vi "PH_ForceSensor.ProcEvents.vi"(0 "i ref in":refnum<vi>, 5 "error in (no error)":errorcluster) -> (14 "i ref out":refnum<vi>, 19 "error out":errorcluster)   [LabVIEW 2014, in "PH_ForceSensor.lvlib"]
doc: "This method is used to define the events the object will listen to. Add your own events here."
uses:
  PH_ForceSensor.lvlib
  CSCore/BaseProcess/BaseProcess.event definition.ctl
  CSCore/CAEObj/CAEObj.event definition.ctl
  CSCore/BaseProcess/BaseProcess.descriptor string definition.ctl
  PH_Beckhoff_StepMot/PH_Beckhoff_StepMot.Force Sensor Tags.ctl
  PH_Beckhoff_StepMot/PH_Beckhoff_StepMot.Force Sensor Location.ctl
  CSCore/BaseProcess/BaseProcess.lvlib
  CSCore/CAEObj/CAEObj.lvlib
  PH_Common/PH_Common.lvlib
  PH_Beckhoff_StepMot/PH_Beckhoff_StepMot.lvlib
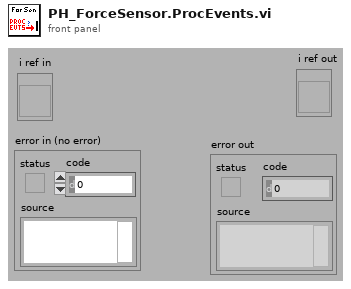
[diagram p1: front panel]
types:
  T1 = typedef "BaseProcess.lvlib/BaseProcess.event definition.ctl" = cluster{"CAEEvtDef":T2, "Data Descriptor":T3}
  T2 = typedef "CAEObj.lvlib/CAEObj.event definition.ctl" = cluster{"URL":string, "enable":bool, "ignoreResID":bool}
  T3 = typedef "BaseProcess.lvlib/BaseProcess.descriptor string definition.ctl" = string
  T4 = typedef "PH_Beckhoff_StepMot.lvlib/PH_Beckhoff_StepMot.Force Sensor Location.ctl" = enum16{"no Info", "MM1"}
  T5 = typedef "PH_Beckhoff_StepMot.lvlib/PH_Beckhoff_StepMot.Force Sensor Tags.ctl" = enum16{"top-front", "top-back", "bottom-front", "bottom-back"}
  T6 = typedef "PH_Common.lvlib/PH_DIM.Event Declarer.ctl" = cluster{"Service Name":string, "Selector":string}
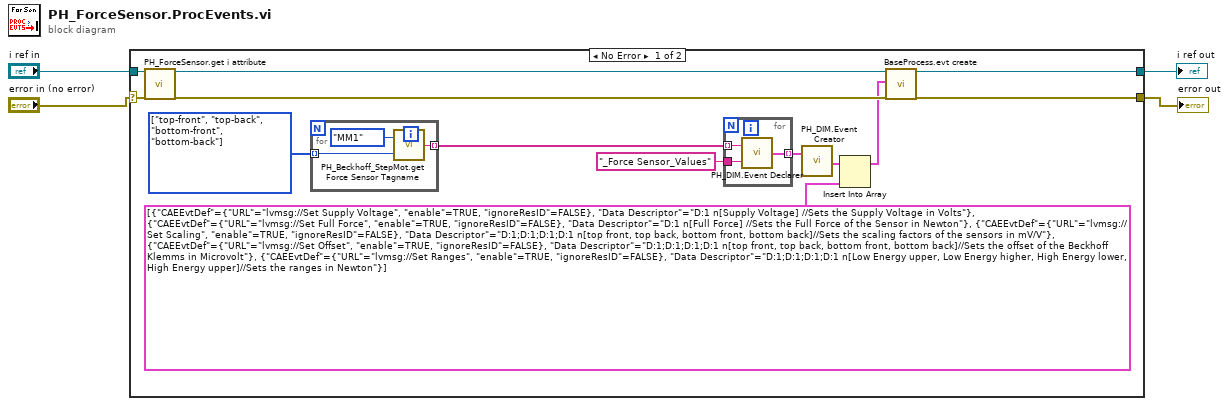
[diagram p0: block diagram]
diagram:
  n1 = case shown="No Error" "error in (no error)" {
    selector: "error in (no error)" -> [w9 w24]
    tunnel: "i ref in" -> [w17 w25]
    tunnel: [w14 w24] -> w3
    tunnel: [w13 w25] -> w2
    frame No Error {
      w7 = T5[] [enum."top-front", enum."top-back", enum."bottom-front", enum."bottom-back"] items=["top-front", "top-back", "bottom-front", "bottom-back"]
      n2 = call "PH_ForceSensor.get i attribute.vi"("i ref in"=w17, "error in (no error)"=w9) -> ("i ref out"=w15:refnum<vi>, "error out"=w16:errorcluster)  [unwired: 15 in, 1 out]
      n3 = for {
        tunnel: w7 -> [w20] mode=indexing
        tunnel: [w18] -> w6 mode=indexing
        n4 = call "PH_Beckhoff_StepMot.get Force Sensor Tagname.vi"("Force Sensor Tag"=w20, "Force Sensor Location"=PH_Beckhoff_StepMot.Force_Sensor_Location."MM1") -> ("Force Sensor Tagname"=w18:string)
      }
      n5 = for {
        tunnel: [w23] -> w12 mode=indexing
        tunnel: "_Force Sensor_Values" -> [w22]
        tunnel: w6 -> [w21] mode=indexing
        n6 = call "PH_DIM.Event Declarer.vi"("Selector"=w22, "Service Name"=w21) -> ("declared DIM Event"=w23:T6)
      }
      n7 = call "PH_DIM.Event Creator.vi"("Trendmessage Services"=w12) -> ("DIM Service Events"=w11:T1[])  [unwired: 18 in]
      n8 = Insert Into Array(array=w11, new element=T1[] [{"CAEEvtDef"={"URL"="lvmsg://Set Supply Voltage", "enable"=TRUE, "ignoreResID"=FALSE}, "Data Descriptor"="D:1 n[Supply Voltage] //Sets the Supply Voltage in Volts"}, {"CAEEvtDef"={"URL"="lvmsg://Set Full Force", "enable"=TRUE, "ignoreResID"=FALSE}, "Data Descriptor"="D:1 n[Full Force] //Sets the Full Force of the Sensor in Newton"}, {"CAEEvtDef"={"URL"="lvmsg://Set Scaling", "enable"=TRUE, "ignoreResID"=FALSE}, "Data Descriptor"="D:1;D:1;D:1;D:1 n[top front, top back, bottom front, bottom back]//Sets the scaling factors of the sensors in mV/V"}, {"CAEEvtDef"={"URL"="lvmsg://Set Offset", "enable"=TRUE, "ignoreResID"=FALSE}, "Data Descriptor"="D:1;D:1;D:1;D:1 n[top front, top back, bottom front, bottom back]//Sets the offset of the Beckhoff Klemms in Microvolt"}, {"CAEEvtDef"={"URL"="lvmsg://Set Ranges", "enable"=TRUE, "ignoreResID"=FALSE}, "Data Descriptor"="D:1;D:1;D:1;D:1 n[Low Energy upper, Low Energy higher, High Energy lower, High Energy upper]//Sets the ranges in Newton"}] ("new events")) -> (w10:T1[])  [unwired: 1 in]
      n9 = call "BaseProcess.evt create.vi"("i ref in"=w15, "newEvents"=w10, "error in (no error)"=w16) -> ("i ref out"=w13:refnum<vi>, "error out"=w14:errorcluster)  [unwired: 13 in, 2 out]
    }
    frame Error {
    }
  }
  "i ref out" <- w2
  "error out" <- w3
